vi "UHR-Fleezers Control (host) - 12.5.vi"() -> ()   [LabVIEW 2012] (continued)
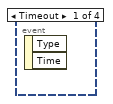
[diagram p2: hidden frame]
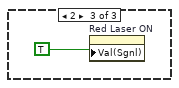
[diagram p5: hidden frame]
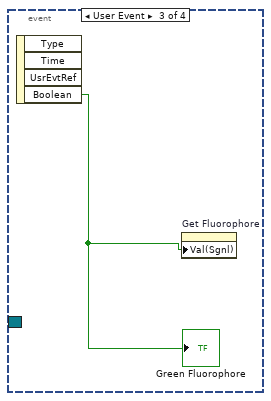
[diagram p6: hidden frame]
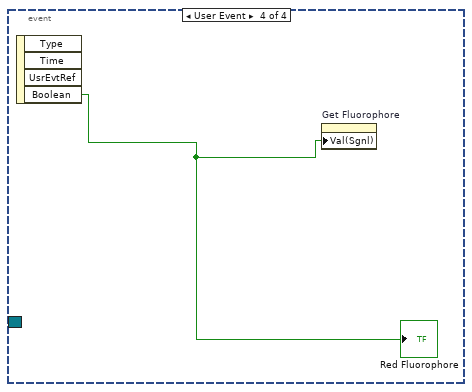
[diagram p7: hidden frame]
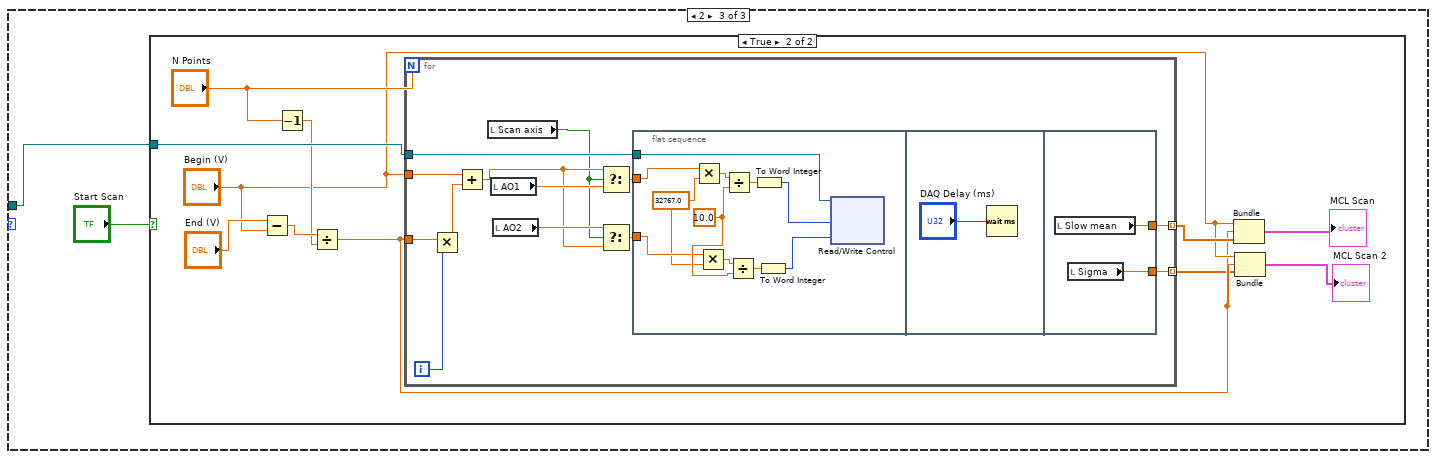
[diagram p9: hidden frame]
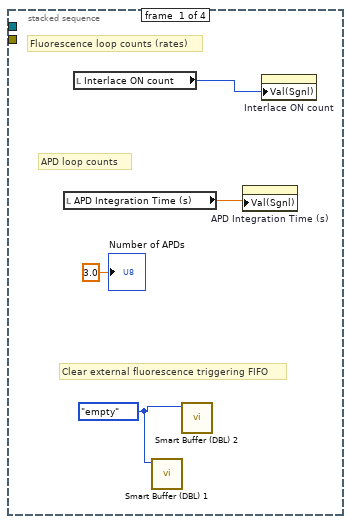
[diagram p11: hidden frame]
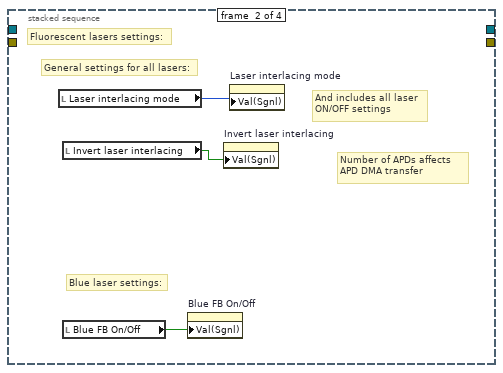
[diagram p12: hidden frame]
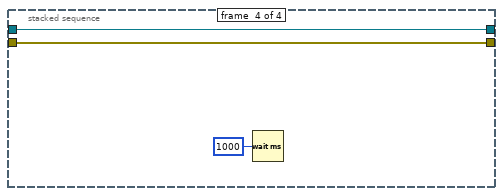
[diagram p13: hidden frame]
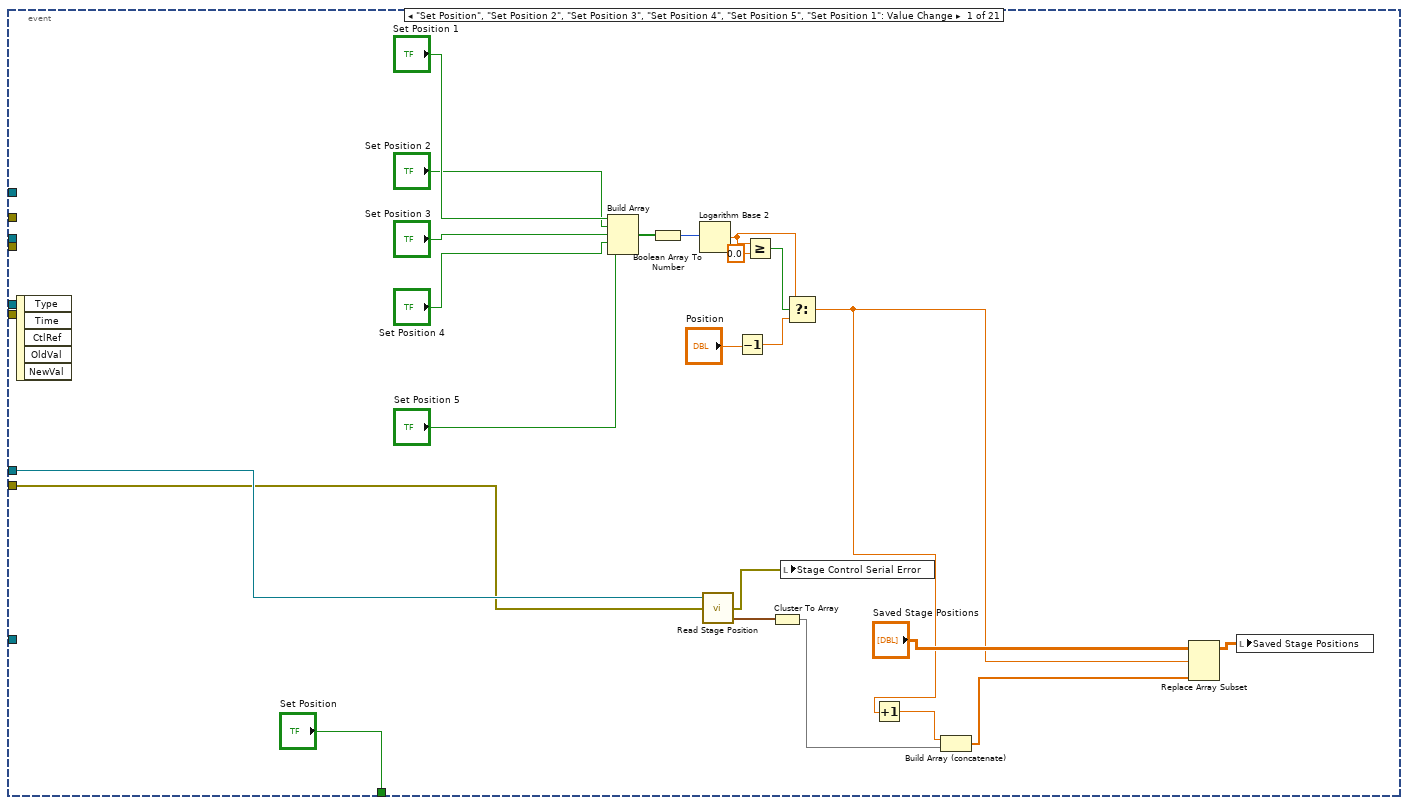
[diagram p15: hidden frame]
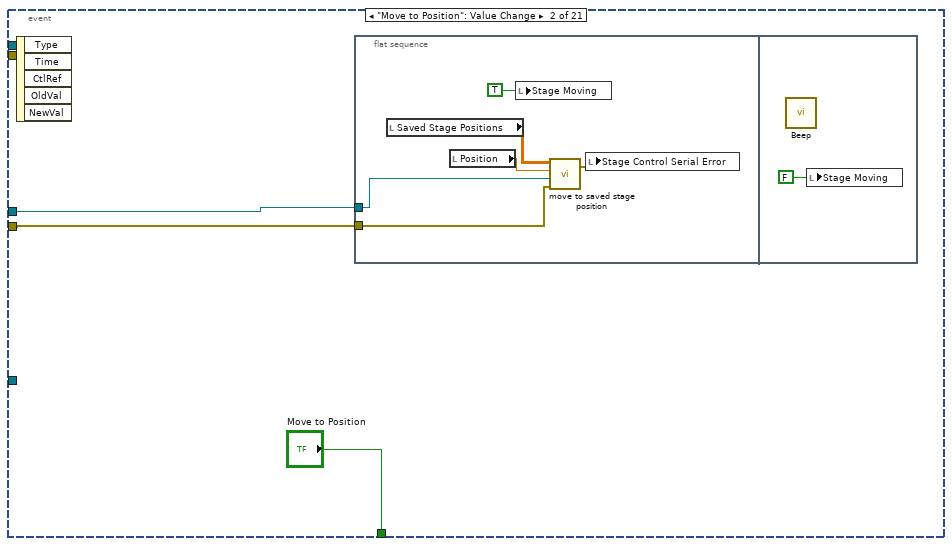
[diagram p16: hidden frame]
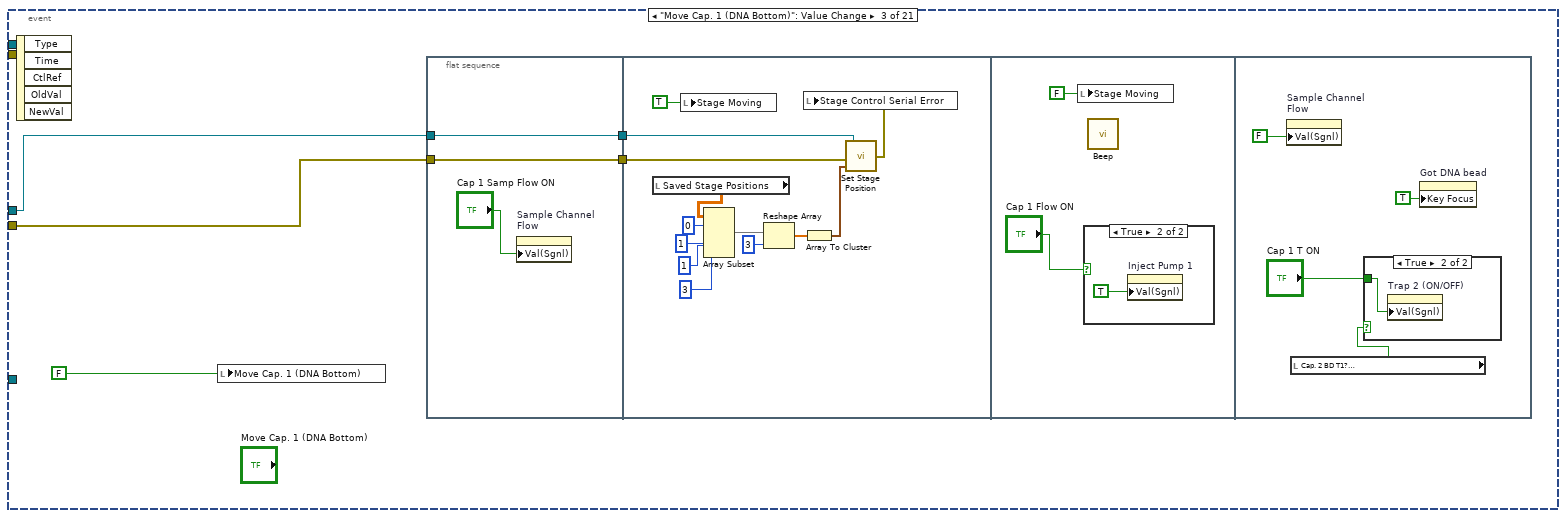
[diagram p17: hidden frame]
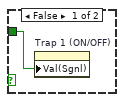
[diagram p19: hidden frame]
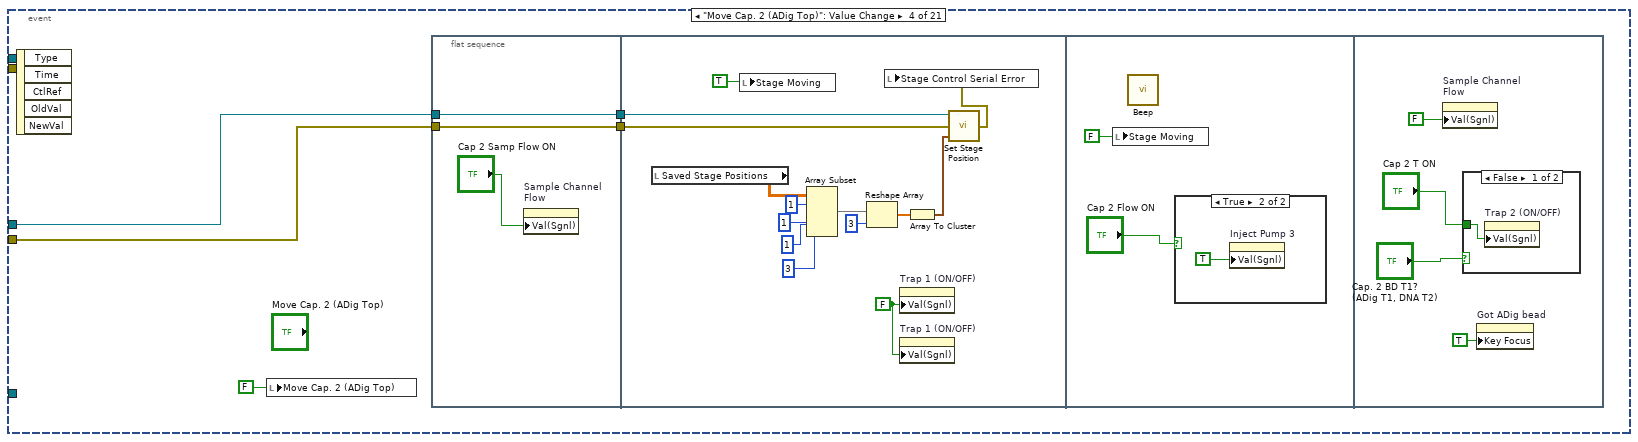
[diagram p20: hidden frame]
              n3244 = Select(t=w5140, s=w5134, f=w5142) -> (s? t:f=w5139:dbl)
              n3245 = Select(t=w5141, s=w5134, f=w5140) -> (s? t:f=w5138:dbl)
              n3246 = flat-sequence {
                tunnel: w5139 -> [w5149]
                tunnel: w5138 -> [w5148]
                tunnel: w5137 -> [w5146]
                tunnel: [w5159] -> w5136
                tunnel: [w5158] -> w5133
                frame #0 {
                  w5152 = 10.0 ("y")
                  w5147 = 32767.0 ("y")
                  n3247 = Multiply(x=w5149, y=w5147) -> (x*y=w5155:dbl)
                  n3248 = Multiply(x=w5148, y=w5147) -> (x*y=w5153:dbl)
                  n3249 = Divide(x=w5155, y=w5152) -> (x/y=w5156:dbl)
                  n3250 = Divide(x=w5153, y=w5152) -> (x/y=w5154:dbl)
                  n3251 = To Word Integer(number=w5156) -> (16bit integer=w5150:i16)
                  n3252 = To Word Integer(number=w5154) -> (16bit integer=w5151:i16)
                  n3253 = xnode "Read/Write Control"("FPGA VI Reference In"=w5146, "AO1"=w5150, "AO2"=w5151) -> ()  [unwired: 1 in, 2 out]
                }
                frame #1 {
                  n3254 = Wait (ms)(milliseconds to wait="DAQ Delay (ms)") -> ()  [unwired: 1 out]
                }
                frame #2 {
                  n3255 = local read "Slow mean"() -> (w5159:dbl)
                  n3256 = local read "Sigma"() -> (w5158:dbl)
                }
              }
            }
            n3257 = Bundle("Begin (V)"="Begin (V)", w5125, w5131) -> (→"MCL Scan":cluster{"Begin (V)":dbl, dbl, dbl[]})  [unwired: 1 out]
            n3258 = Bundle("Begin (V)"="Begin (V)", w5125, w5124) -> (→"MCL Scan 2":cluster{"Begin (V)":dbl, dbl, dbl[]})  [unwired: 1 out]
          }
        }
      }
    }
    n3259 = local read "Stop All"() -> (w5069:bool)
    n3260 = node-c288() -> ()  [unwired: 2 out]
  }
  n3261 = node-c288(w6) -> ()  [unwired: 1 out]
  n3262 = node-c288(w126) -> ()  [unwired: 1 out]
  n3263 = node-c288(w128) -> ()  [unwired: 1 out]
  n3264 = property on="Saved trap pos" class="WFGraph (strict)"("Visible"=FALSE) -> ()  [unwired: 2 in, 2 out]
  n3265 = property on="Trap Delta Graph" class="WFGraph (strict)"("Visible"=TRUE) -> ()  [unwired: 2 in, 2 out]
  n3266 = node-c288(w113) -> ()  [unwired: 1 out]
  n3267 = local write "Trap pos"(FALSE ("Trap pos")) -> ()
  n3268 = disable-structure shown="Disabled" {
    disable-tunnel: w117 -> [w5161 _]
    disable-tunnel: w116 -> [w5160 _]
    frame Disabled {
      n3269 = VISA Close(VISA resource name=w5161, error in (no error)=w5160) -> (error out=w5162:errorcluster)
      n3270 = call <vilib>:"Simple Error Handler.vi"("error in (no error)"=w5162) -> ()  [unwired: 1 in, 8 out]
    }
    frame Enabled {
    }
  }
  n3271 = node-c288(w199) -> ()  [unwired: 1 out]
  n3272 = node-c288(w124) -> ()  [unwired: 1 out]
  n3273 = flat-sequence {
    tunnel: w290 -> [w5166]
    tunnel: w292 -> [w5167]
    tunnel: [w5165] -> w271
    tunnel: [w5164] -> w270
    tunnel: w255 -> [_]
    tunnel: w207 -> [_]
    tunnel: w130 -> [_]
    tunnel: w271 -> [w5168]
    tunnel: w270 -> [w5169]
    frame #0 {
      w5163 = FALSE ("AI to FIFO")
      n3274 = xnode "Read/Write Control"("FPGA VI Reference In"=w5167, "error in"=w5166, "AI to FIFO"=w5163, "APD to FIFO"=w5163) -> ("FPGA VI Reference Out"=w5165:T20, "error out"=w5164:errorcluster)
    }
    frame #1 {
      n3275 = xnode "Close FPGA VI Reference"("FPGA VI Reference In"=w5168, "error in"=w5169) -> ("error out"=→"error out":errorcluster)
    }
  }
